vi "Acknowledge Alarm.vi"(7 "Unit Address (1)":u8=1, 8 "error in (no error)":errorcluster, 9 "Enable Alarm Group (True)":bool=TRUE, 10 "Alarm Number (1)":u16=1 min=1 max=8, 11 "VISA resource name":refnum<visa-resource-name>) -> (0 "error out":errorcluster, 3 "VISA resource name out":refnum<visa-resource-name>)   [LabVIEW 2014, in "Eurotherm 35xx Series.lvlib"]
doc: "This VI acknowledge selected alarm."
uses:
  <instrlib>/Eurotherm 35xx Series/Eurotherm 35xx Series.lvlib
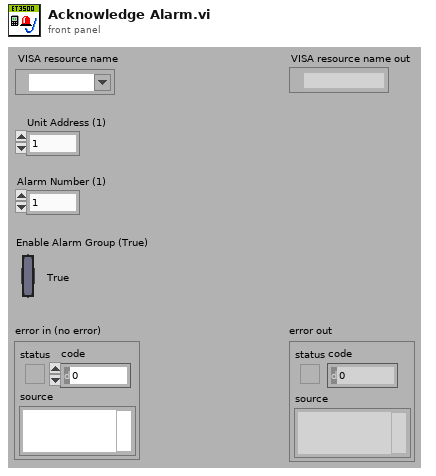
[diagram p1: front panel]
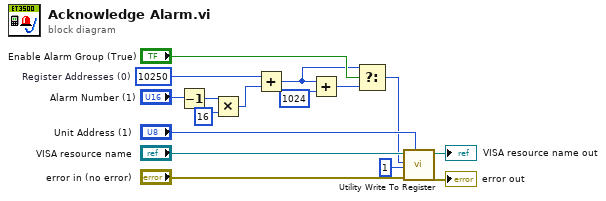
[diagram p0: block diagram]
diagram:
  w12 = 10250  # Register Addresses (0)
  n1 = Decrement(x="Alarm Number (1)") -> (x-1=w15:u16)
  n2 = Multiply(x=w15, y=u16 16) -> (x*y=w13:u16)
  n3 = Add(x=w12, y=w13) -> (x+y=w8:i32)
  n4 = Add(x=w8, y=1024) -> (x+y=w9:i32)
  n5 = Select(t=w8, s="Enable Alarm Group (True)", f=w9) -> (s? t:f=w2:i32)
  n6 = call <instrlib>:"Utility Write To Register.vi"("Unit Address (1)"="Unit Address (1)", "error in (no error)"="error in (no error)", "Data (0)"=i16 1, "Register Address (0)"=w2, "VISA resource name"="VISA resource name") -> ("error out"=→"error out":errorcluster, "VISA resource name out"=→"VISA resource name out":refnum<visa-resource-name>)  [unwired: 5 in]
